vi "דף פתיחה עם תמונות 8.11.vi"() -> ()   [LabVIEW 2013]
uses:
  <vilib>/picture/picture.llb/imagedata.ctl
  <vilib>/Utility/miscctls.llb/LVBoundsTypeDef.ctl
panel:
  in  "stop":bool
  in  "enter system":bool
  out "image data":T1
  out "Array":path[](array[path])
  out "new picture":picture
  # "Fider"
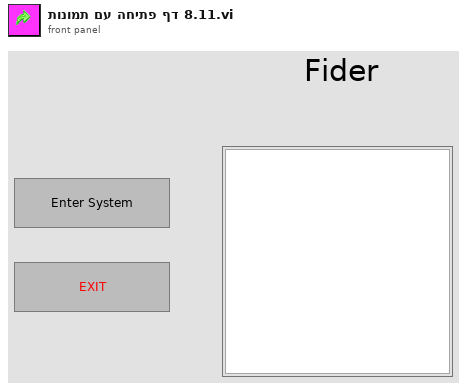
[diagram p1: front panel]
types:
  T1 = typedef "imagedata.ctl" = cluster{"image type":i32, "image depth":i32, "image":u8[], "mask":u8[], "colors":u32[], "Rectangle":cluster{"left":i16, "top":i16, "right":i16, "bottom":i16}}
  T2 = typedef "LVBoundsTypeDef.ctl" = cluster{"Width":u32, "Height":u32}
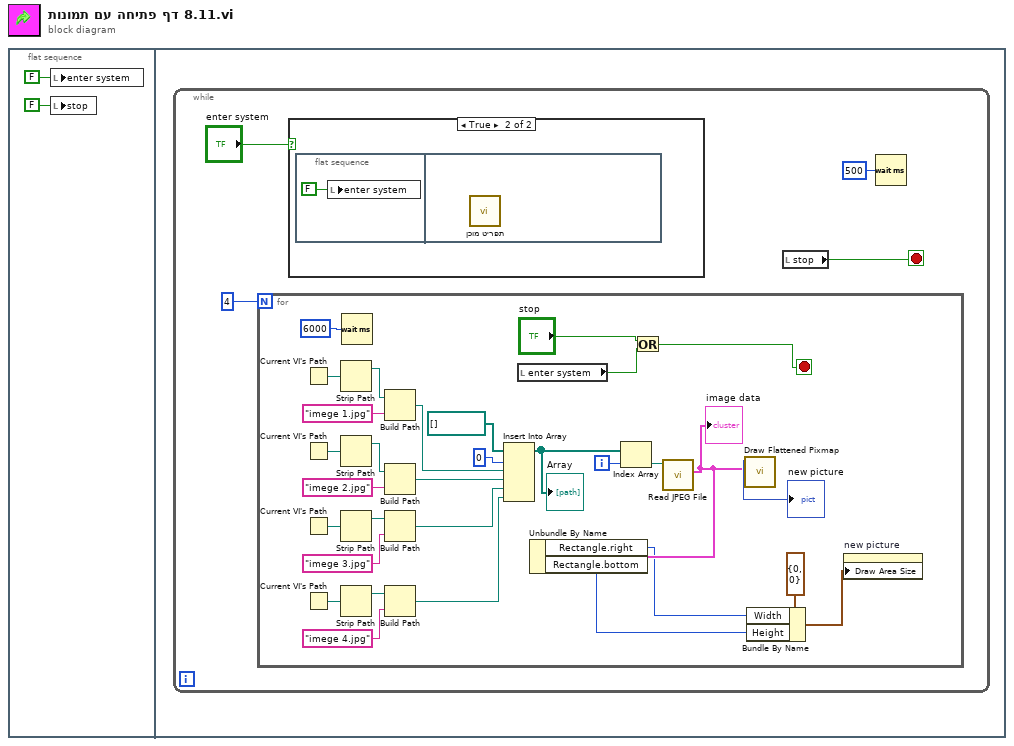
[diagram p0: block diagram]
diagram:
  n1 = flat-sequence {
    frame #0 {
      n2 = local write "enter system"(FALSE ("OK Button")) -> ()
      n3 = local write "stop"(FALSE ("stop")) -> ()
    }
    frame #1 {
      n4 = while {
        stop <- w3 stop-if-true
        n5 = for {
          N: 4 -> [_]
          i -> [w32]
          stop <- w8 stop-if-true
          n6 = Current VI's Path() -> (path=w28:path)
          n7 = Current VI's Path() -> (path=w29:path)
          n8 = Current VI's Path() -> (path=w30:path)
          n9 = Current VI's Path() -> (path=w31:path)
          n10 = Strip Path(path=w28) -> (stripped path=w23:path)  [unwired: 1 out]
          n11 = Strip Path(path=w29) -> (stripped path=w22:path)  [unwired: 1 out]
          n12 = Strip Path(path=w30) -> (stripped path=w21:path)  [unwired: 1 out]
          n13 = Strip Path(path=w31) -> (stripped path=w20:path)  [unwired: 1 out]
          n14 = Wait (ms)(milliseconds to wait=u32 6000) -> ()  [unwired: 1 out]
          n15 = Build Path(base path=w23, name or relative path="imege 1.jpg") -> (appended path=w26:path)
          n16 = Build Path(base path=w22, name or relative path="imege 2.jpg") -> (appended path=w25:path)
          n17 = Build Path(base path=w21, name or relative path="imege 3.jpg") -> (appended path=w24:path)
          n18 = Build Path(base path=w20, name or relative path="imege 4.jpg") -> (appended path=w27:path)
          n19 = Insert Into Array(array=path[] [], index=0, new element #1=w26, new element #2=w25, new element #3=w24, new element #4=w27) -> (w36:path[])
          "Array" <- w36
          n20 = local read "enter system"() -> (w9:bool)
          n21 = Index Array(array=w36, index=w32) -> (element=w37:path)
          n22 = Or(x="stop", y=w9) -> (x .or. y?=w8:bool)
          n23 = call <vilib>:"Read JPEG File.vi"("path to JPEG file"=w37) -> ("image data"=w13:T1)  [unwired: 8 in, 2 out]
          "image data" <- w13
          n24 = Unbundle By Name(w13) -> ("Rectangle.right"=w12:i16, "Rectangle.bottom"=w11:i16)
          n25 = call <vilib>:"Draw Flattened Pixmap.vi"("image data"=w13) -> ("new picture"=→"new picture":picture)  [unwired: 8 in]
          n26 = Bundle By Name(cluster=T2 {"Width"=0, "Height"=0} ("Draw Area Size"), "Width"=w12, "Height"=w11) -> (w14:T2)
          n27 = property on="new picture" class="Pict"("Draw Area Size"=w14) -> ()  [unwired: 2 in, 2 out]
        }
        n28 = case shown="True" "enter system" {
          frame False {
          }
          frame True {
            n29 = flat-sequence {
              frame #0 {
                n30 = local write "enter system"(FALSE ("OK Button")) -> ()
              }
              frame #1 {
                n31 = call "תפריט מוכן.vi"() -> ()  [unwired: 1 in]
              }
            }
          }
        }
        n32 = local read "stop"() -> (w3:bool)
        n33 = Wait (ms)(milliseconds to wait=u32 500) -> ()  [unwired: 1 out]
      }
    }
  }
